vi "LabVIEW Error.vi"(11 "ErrorOrSuccess in":refnum<class "ErrorOrSuccess.lvclass">) -> (2 "Associated LabVIEW Error":errorcluster, 3 "ErrorOrSuccess out":refnum<class "ErrorOrSuccess.lvclass">)   [LabVIEW 2020, in "wamplv.lvlib" / "ErrorOrSuccess.lvclass"]
uses:
  ErrorOrSuccess.lvclass
  ErrorOrSuccess.lvclass/ErrorOrSuccess.ctl
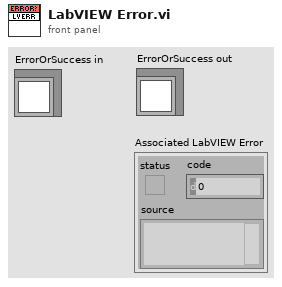
[diagram p1: front panel]
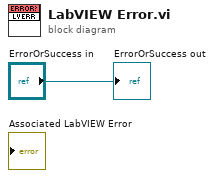
[diagram p0: block diagram]
diagram:
  "ErrorOrSuccess out" <- "ErrorOrSuccess in"
